vi "Helper SubVI - Wrap to Power of 2.vi"(6 "low constraint":i32, 7 "default":i32=512, 8 "where to go":u16(ring) items=["nearest", "lower", "upper"], 9 "power of 2":bool=TRUE, 11 "number in":i32) -> (3 "number out":i32)   [LabVIEW 2023]
doc: "Rounds the input to the nearest, next lowest, or next highest power of 2."
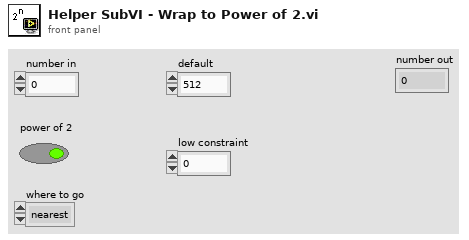
[diagram p1: front panel]
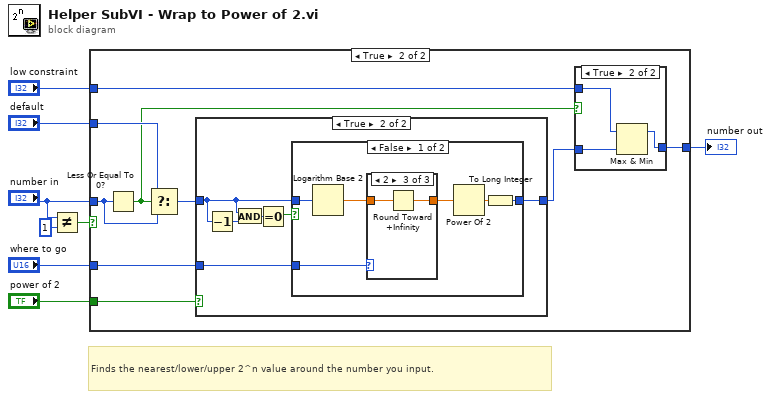
[diagram p0: block diagram]
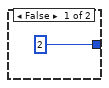
[diagram p2: hidden frame]
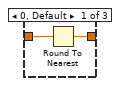
[diagram p5: hidden frame]
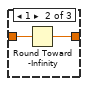
[diagram p6: hidden frame]
diagram:
  # "Finds the nearest/lower/upper 2^n value around the number you input."
  n1 = Not Equal?(x="number in", y=1) -> (x != y?=w4:bool)
  n2 = case shown="True" w4 {
    tunnel: "default" -> [_ w18]
    tunnel: "power of 2" -> [_ w17]
    tunnel: "number in" -> [_ w16]
    tunnel: [2 w13] -> w6
    tunnel: "where to go" -> [_ w11]
    tunnel: "low constraint" -> [_ w10]
    frame False {
    }
    frame True {
      n3 = Less Or Equal To 0?(x=w16) -> (x <= 0?=w12:bool)
      n4 = Select(t=w18, s=w12, f=w16) -> (s? t:f=w15:i32)
      n5 = case shown="True" w17 {
        tunnel: [w23 w25] -> w14
        tunnel: w15 -> [w23 w28]
        tunnel: w11 -> [_ w24]
        frame False {
        }
        frame True {
          n6 = Decrement(x=w28) -> (x-1=w29:i32)
          n7 = And(x=w28, y=w29) -> (x .and. y?=w27:i32)
          n8 = Equal To 0?(x=w27) -> (x = 0?=w26:bool)
          n9 = case shown="False" w26 {
            tunnel: [w35 w42] -> w25
            tunnel: w28 -> [w33 w42]
            tunnel: w24 -> [w30 _]
            frame False {
              n10 = Logarithm Base 2(1:w33) -> (0:w32:dbl)
              n11 = case shown="2" w30 {
                tunnel: w32 -> [w37 w39 w41]
                tunnel: [w36 w38 w40] -> w31
                frame 0, Default {
                  n12 = Round To Nearest(number=w37) -> (nearest integer value=w36:dbl)
                }
                frame 1 {
                  n13 = Round Toward -Infinity(1:w39) -> (0:w38:dbl)
                }
                frame 2 {
                  n14 = Round Toward +Infinity(x=w41) -> (ceil(x): smallest int >= x=w40:dbl)
                }
              }
              n15 = Power Of 2(x=w31) -> (2^x=w34:dbl)
              n16 = To Long Integer(number=w34) -> (32bit integer=w35:i32)
            }
            frame True {
            }
          }
        }
      }
      n17 = case shown="True" w12 {
        tunnel: w14 -> [w19 w22]
        tunnel: [w19 w21] -> w13
        tunnel: w10 -> [_ w20]
        frame False {
        }
        frame True {
          n18 = Max & Min(x=w20, y=w22) -> (max(x,y)=w21:i32)  [unwired: 1 out]
        }
      }
    }
  }
  "number out" <- w6
